vi "Text control 2 v0.7.vi"() -> ()   [LabVIEW 2016]
panel:
  out "error out":errorcluster
  in  "Units":bool
  out "Elapsed Time":dbl caption="Elapsed Time (s)"
  out "Ion vs time":cluster{"Y data in":dbl[], "X data in":dbl[]}[](graph)
  out "Ig":dbl format="%.2e"
  out "Id":dbl format="%.2e"
  out "Is":dbl format="%.2e"
  out "I vs Vg":cluster{"Y data in":dbl[], "X data in":dbl[]}[](graph)
  in  "Panel Controls 2":T1={"Emergency Stop"=refnum, "TransGraph Max"=1e-05, "Text/Graph (text=false)"=TRUE, "TransGraph Min"=1e-11} {"TransGraph Min" format="%.2e"; "TransGraph Max" format="%.2e"}
  out "Currently running:":string="#output s 0 0 0 -0.008 0.008 0.002"
  in  "Lines left to run:":string
  in  "Standby":T2
  in  "Full Reset":bool
  in  "SMU4":cluster{"on/off":bool, "Voltage":dbl} {"Voltage" min=-100.0 max=100.0 format="%.2f"}
  in  "Source/Drain Range":u8(slide)=6 max=11 scale=0.0..11.0
  in  "Source/Drain\nRange mode":u16(ring) items=["Auto", "Limited", "Fixed"]
  in  "Gate Range":u8(slide)=6 max=11 scale=0.0..11.0
  in  "Gate Range\nmode":u16(ring) items=["Auto", "Limited", "Fixed"]
  in  "Gate":T3={"Gate Start"=0.0, "Gate Stop"=2.0, "Gate Step (linear only)"=1.0, "Gate Compliance"=0.0001, "Gate PComp"=0.0, "Range mode"=0, "Range"=6} {"Range" max=11 scale=0.0..11.0; "Range mode" items=["Auto", "Limited", "Fixed"]; "Gate PComp" format="%^.2e"; "Gate Compliance" format="%^.2e"; "Gate Step (linear only)" format="%^.4e"; "Gate Stop" format="%^.4e"; "Gate Start" format="%^.4e"}
  in  "Drain 2":T4={"Drain Start"=0.0, "Drain Stop"=2.0, "Drain Compliance"=0.0001, "Drain Step"=1.0, "Drain PComp"=0.0, "Range mode"=0, "Range"=6} {"Range" max=11 scale=0.0..11.0; "Range mode" items=["Auto", "Limited", "Fixed"]; "Drain PComp" format="%^.2e"; "Drain Step" format="%^.4e"; "Drain Compliance" format="%^.2e"; "Drain Stop" format="%^.4e"; "Drain Start" format="%^.4e"}
  in  "Timings 2":T5={"integration time"=0, "Short/Long integration time"=0.00064, "hold time (sec)"=0.0, "delay time (sec)"=0.0, "Step Time (0 disables)"=0.0, "sweep method"=0, "Pulse period"=0.005, "Base voltage"=0.0, "Pulse width"=0.0005} {"Pulse width" min=0.0005 max=0.1 step=0.0001 format="%.4f"; "Base voltage" format="%^.4e"; "Pulse period" min=0.005 max=1.0 step=0.0001 format="%.4f"; "sweep method" items=["Continuous", "Pulsed"]; "Step Time (0 disables)" format="%.2f"; "delay time (sec)" format="%.4f"; "hold time (sec)" format="%.4f"; "Short/Long integration time" format="%^.0e"; "integration time" scale=0.0..2.0}
  in  "Panel Controls":T6={"Emergency Stop"=refnum, "TransGraph Max"=1e-05, "Text/Graph (text=false)"=TRUE} {"TransGraph Max" format="%.2e"}
  in  "Interrupt run":bool
  in  "Drain: Compliance":dbl=0.001 format="%.8f"
  in  "Gate: Compliance":dbl=0.001 format="%.8f"
  out "Path":path=path "C:/users/rlp38/09Apr2009LTtesting/test2.txt"
  in  "hold time /s":dbl format="%.2f"
  in  "delay time /s":dbl format="%.2f"
  in  "integration time":u32(slide) max=2 step=1 scale=0.0..2.0
  in  "Integration time (short)":dbl=0.0019 min=8e-05 max=0.0019 step=8e-05 format="%^.0e"
  in  "Integration time (long)":dbl=0.32 min=0.04 max=2.0 step=0.02 format="%.2f"
  in  "Step delay /s":dbl format="%.2f"
  in  "Program":string="#pulsedstressV d 0.03 20 0 0.5 0.0827 5\n#\nitime s\ngaterangemode l\ndrainrangemode l\n#pulsed on 0.05 0 0.02\ntransfer d 1 -1 -0.1 -1 -1 0\nwait-min 1\ntransfer d 1 -1 -0.1 -1 -1 0\n#transfer d -10 40 1 5 40 35\n#transfer d -10 40 1 5 40 35\n#output d 0 40 20 0 40 1\n#\n#\n#sample 1 0.008 221 6 0.003\n#samplei 400e-6 200 6 0.002 0.1\n#vsu2pulse -10 4\n#\n#stressV 0.016 0.03 2e-4 0.1e-3 11\n#stressI 220e-7 0.08 15\n#transfer s -1 1 0.5 -0.005 0.005 0.005\n#output s 0 0 0 -0.008 0.008 0.002\n"
  # "Syntax:\nitime [s|m|l]\ngaterangemode [a|l|f]\ndrainrangemode [a|l|f]\npulsed [on|off] PulsePeriod(sec) PulseBaseVoltage PulseONWidth(sec)\nstandby [on l off]\nwait NumMilliseconds\nwait-min NumMinutes\n# texthere = comment\ntransfer [s|d] VgStart VgStop VgStep VdStart VdStop VdStep\noutput [s|d] VgStart VgStop VgStep VdStart VdStop VdStep\nsample Vg Vd NumSamples Time(s) SampleInterval(s)\nsamplei Idg NumSamples Time(s) SampleInterval(s) VDGcompliance\n# if in doubt use SampleInterval(s) = 0.004\nstressV VG VD IGcompliance IDcompliance Duration(sec)\nstressI IDG VDGcompliance Duration(sec)\nvsu2pulse Bias Duration(s)\npulsedstressV [s|d] VEstop VgON VgOFF Period(s) PulseONwidth(s) Vd\nsample-fpp Vg Vd NumSamples Time\nresample-fpp Vg Vd\ntransfer-fpp [s|d] VgStart VgStop VgStep VdStart VdStop VdStep\noutput-fpp [s|d] VgStart VgStop VgStep VdStart VdStop VdStep"
  # "Sec"
  # "Min"
  # "100 samples is approx 13s with medium integration"
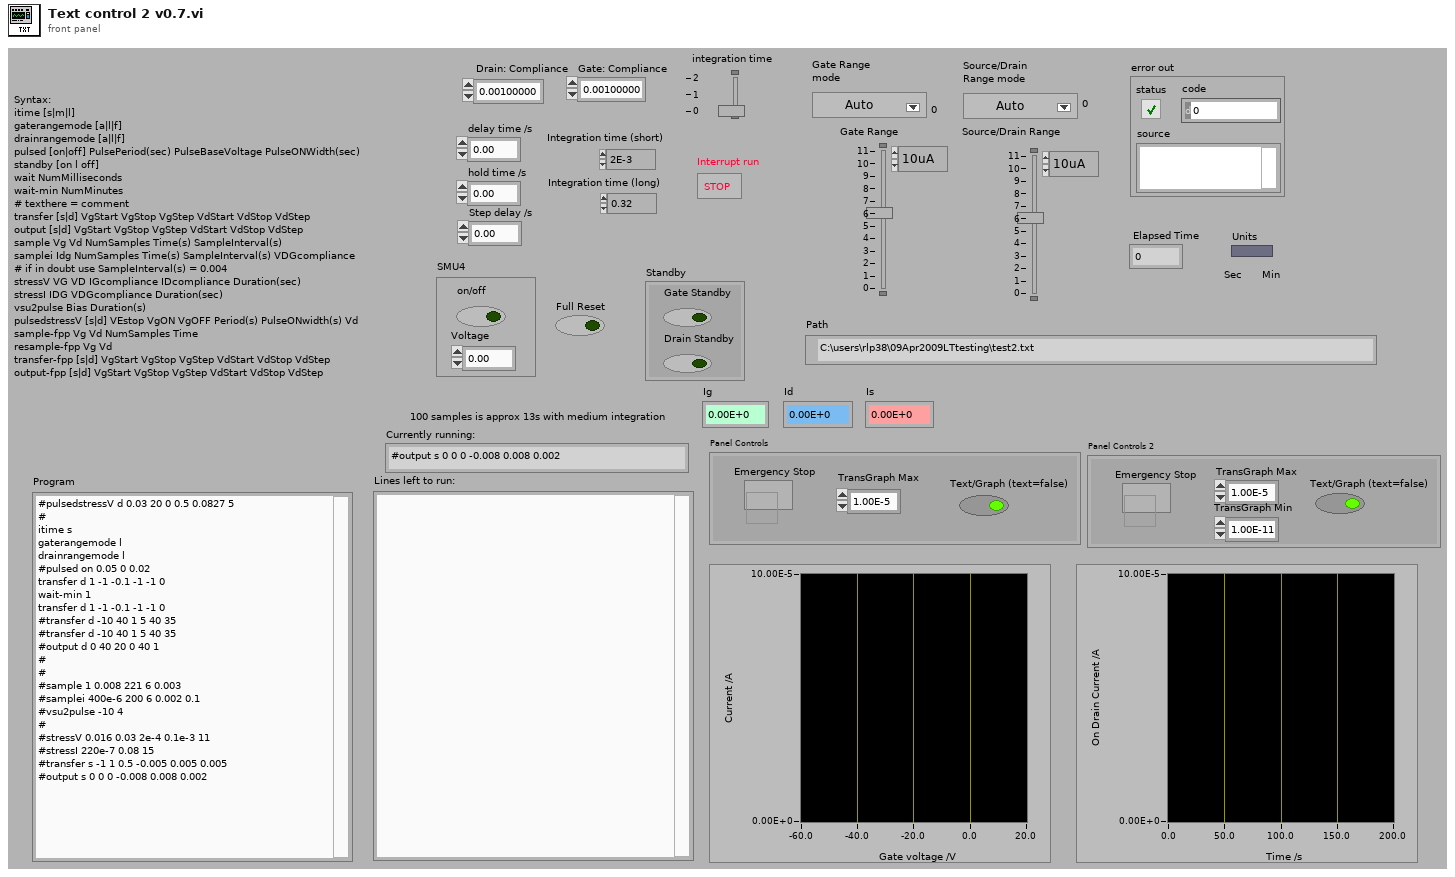
[diagram p1: front panel]
types:
  T1 = cluster{"Emergency Stop":refnum<vi>, "TransGraph Max":dbl, "Text/Graph (text=false)":bool, "TransGraph Min":dbl}
  T2 = cluster{"Gate Standby":bool, "Drain Standby":bool}
  T3 = cluster{"Gate Start":dbl, "Gate Stop":dbl, "Gate Step (linear only)":dbl, "Gate Compliance":dbl, "Gate PComp":dbl, "Range mode":u16, "Range":u8}
  T4 = cluster{"Drain Start":dbl, "Drain Stop":dbl, "Drain Compliance":dbl, "Drain Step":dbl, "Drain PComp":dbl, "Range mode":u16, "Range":u8}
  T5 = cluster{"integration time":u32, "Short/Long integration time":dbl, "hold time (sec)":dbl, "delay time (sec)":dbl, "Step Time (0 disables)":dbl, "sweep method":u16, "Pulse period":dbl, "Base voltage":dbl, "Pulse width":dbl}
  T6 = cluster{"Emergency Stop":refnum<vi>, "TransGraph Max":dbl, "Text/Graph (text=false)":bool}
  T7 = enum16{"open", "replace", "create", "open or create", "replace or create", "replace or create with confirmation"}
  T8 = cluster{"V2 Start":dbl, "V2 Step":dbl, "Number of points":i32}
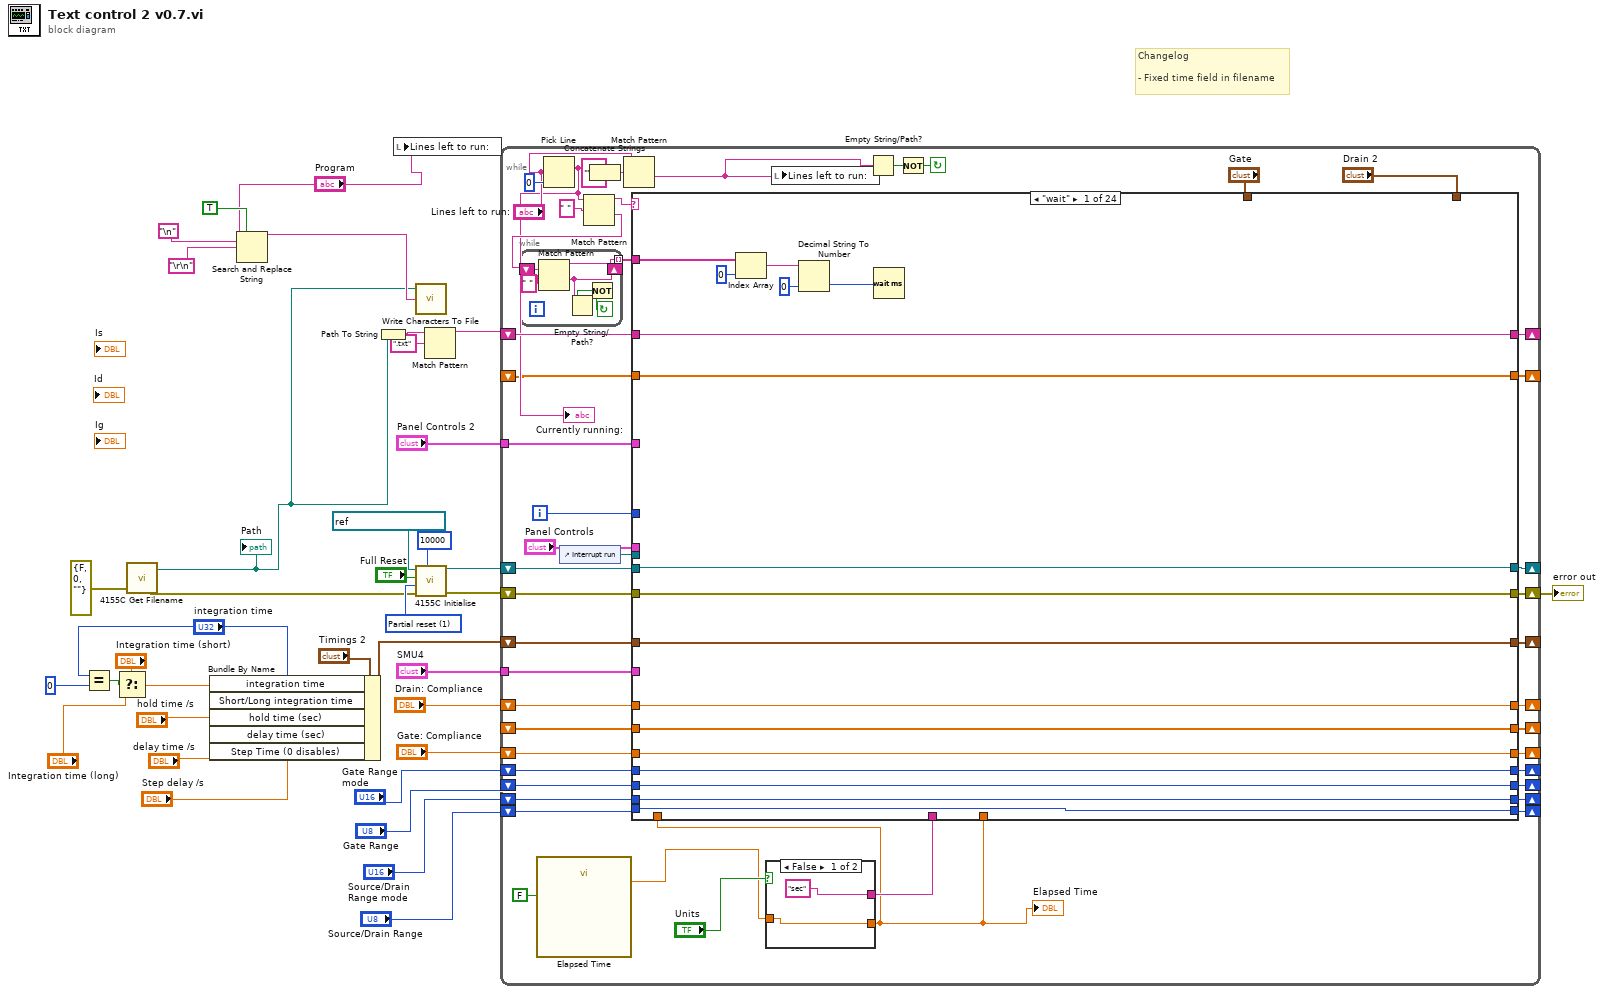
[diagram p0: block diagram]
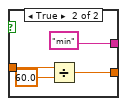
[diagram p2: hidden frame]
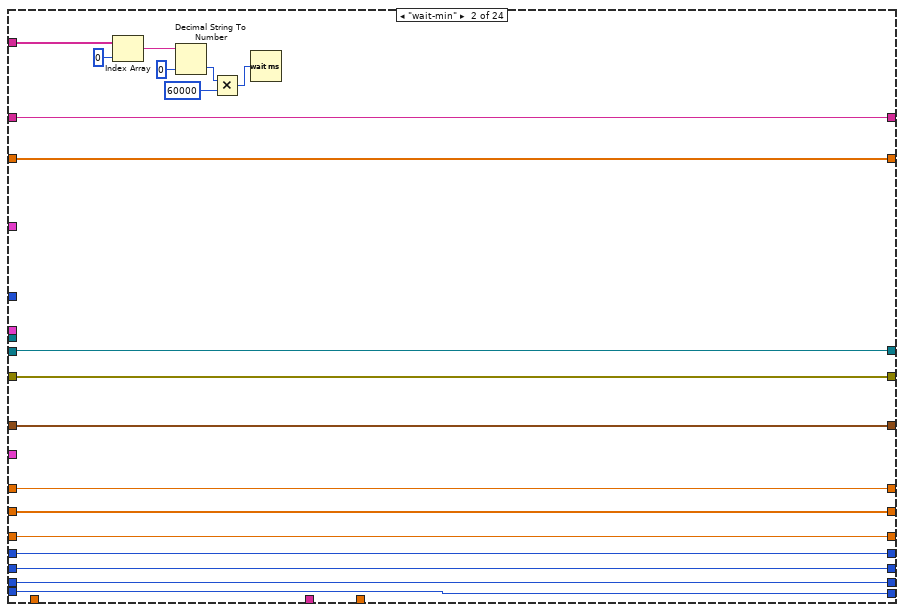
[diagram p3: hidden frame]
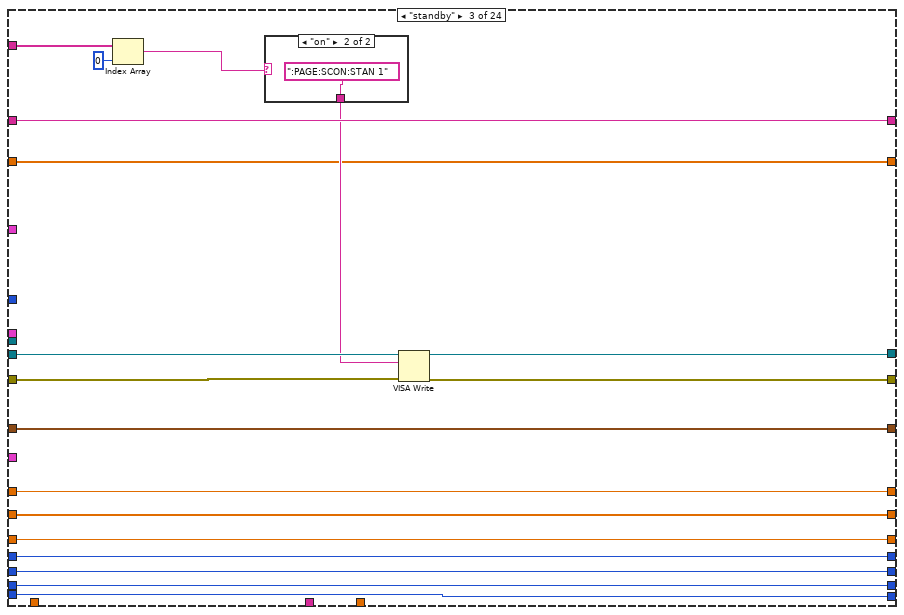
[diagram p4: hidden frame]
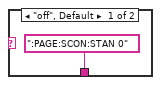
[diagram p5: hidden frame]
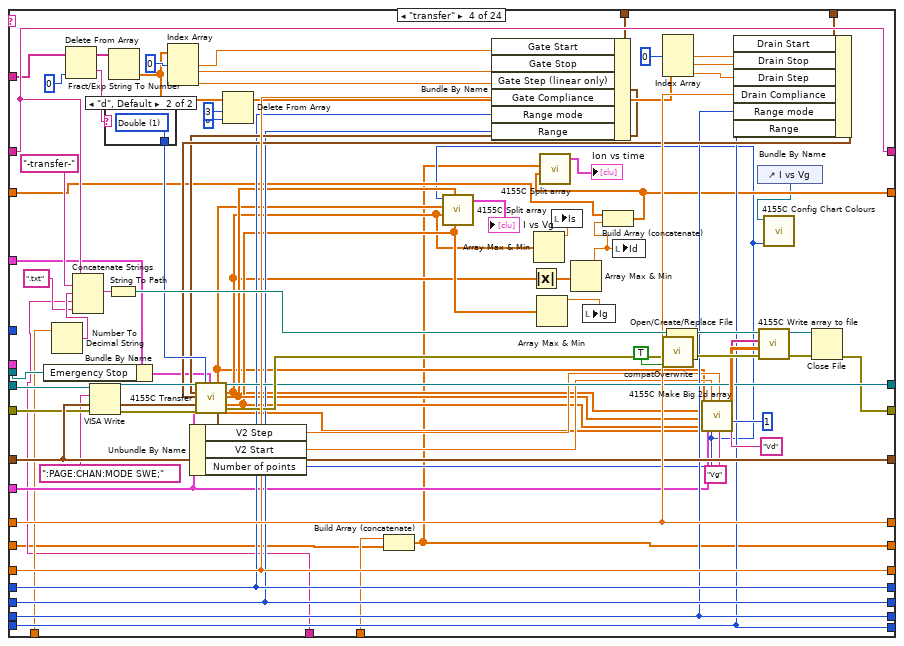
[diagram p6: hidden frame]
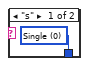
[diagram p7: hidden frame]
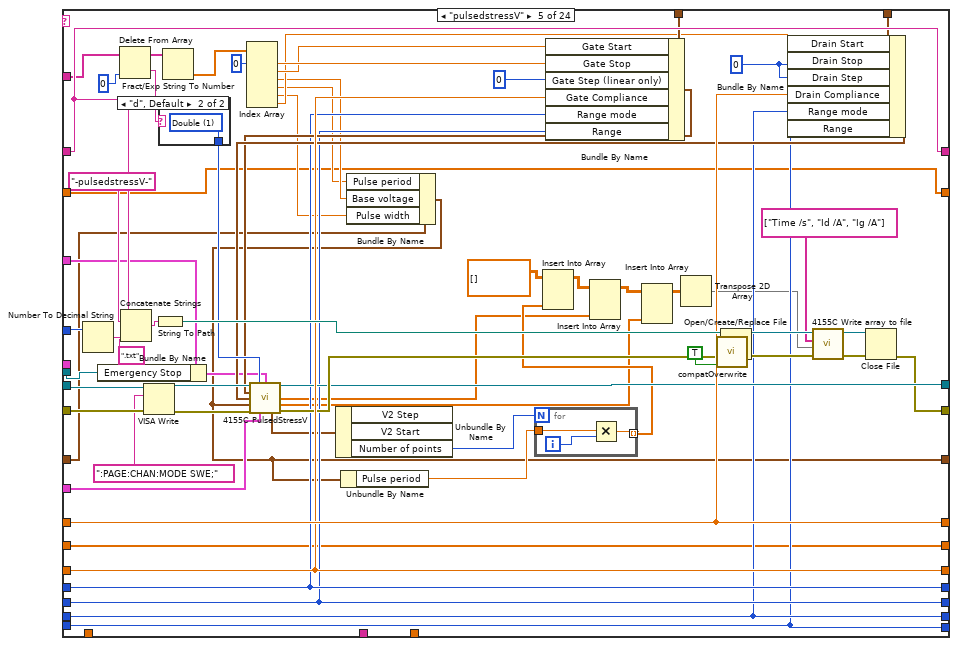
[diagram p8: hidden frame]
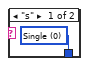
[diagram p9: hidden frame]
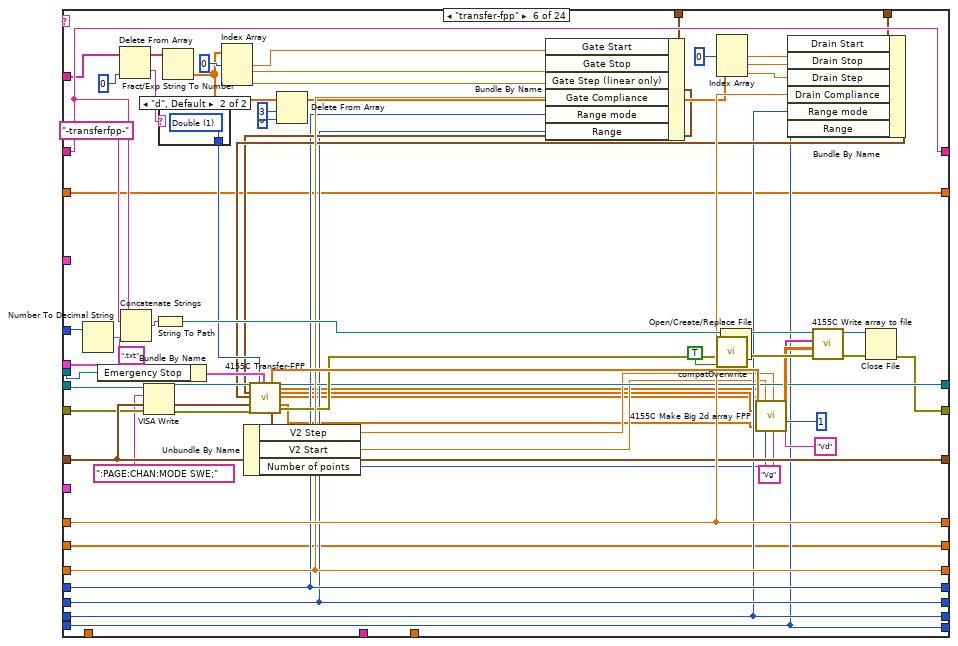
[diagram p10: hidden frame]
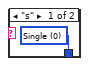
[diagram p11: hidden frame]
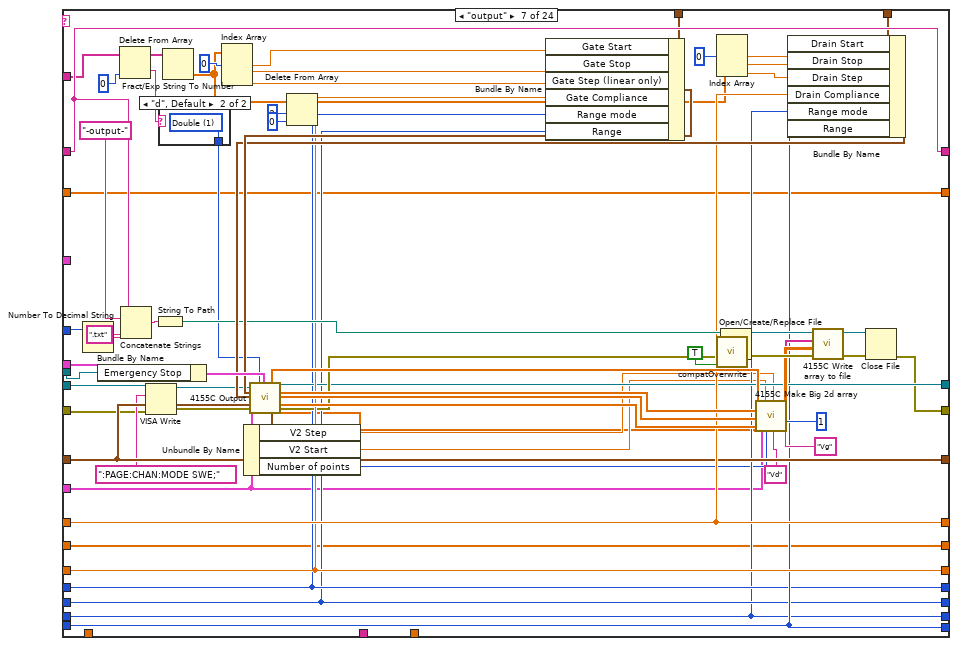
[diagram p12: hidden frame]
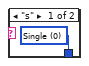
[diagram p13: hidden frame]
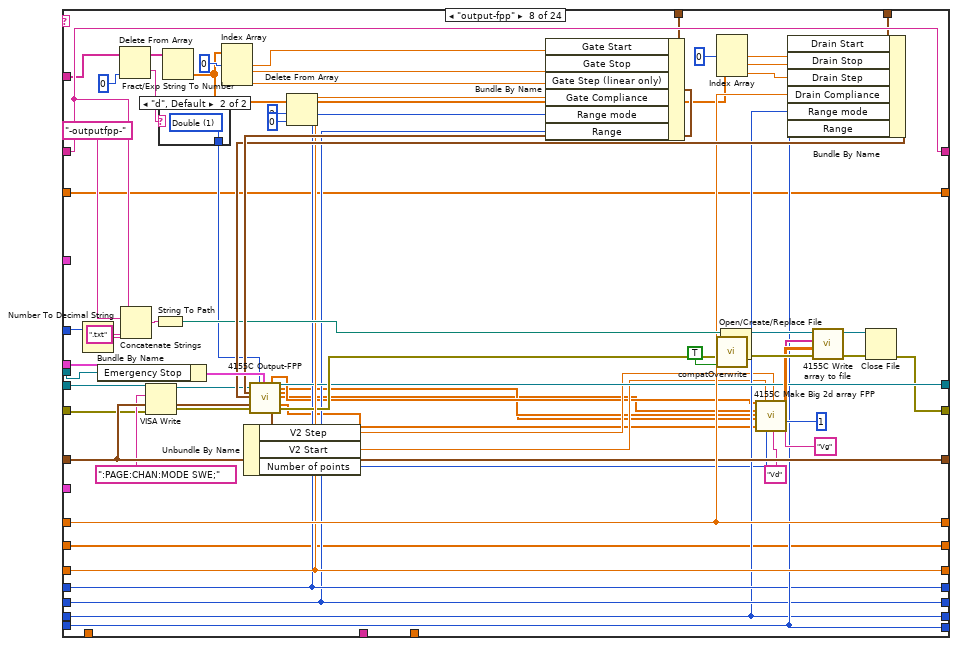
[diagram p14: hidden frame]
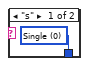
[diagram p15: hidden frame]
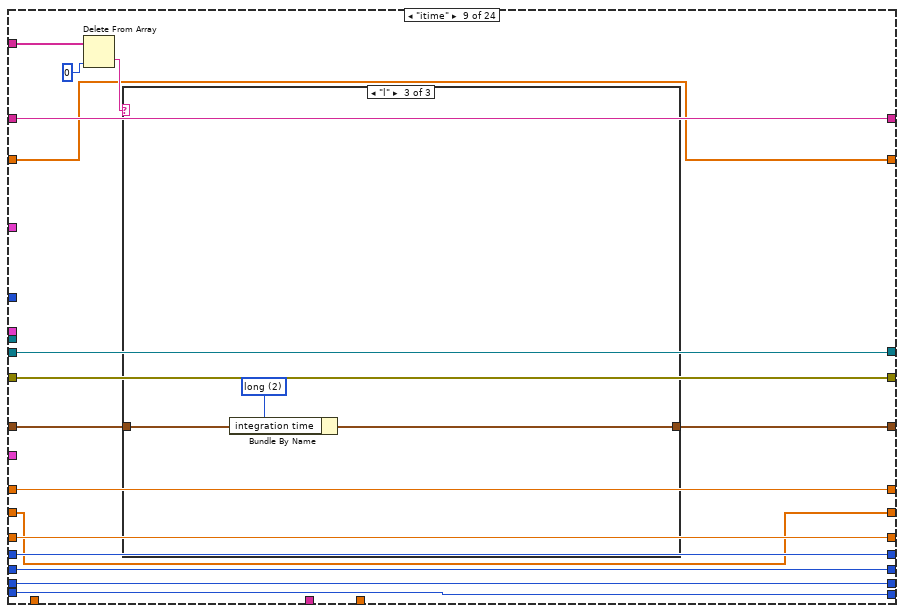
[diagram p16: hidden frame]
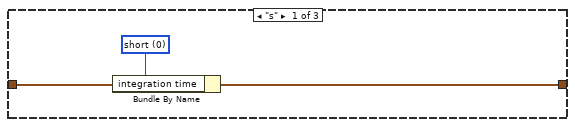
[diagram p17: hidden frame]
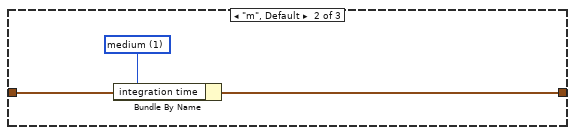
[diagram p18: hidden frame]
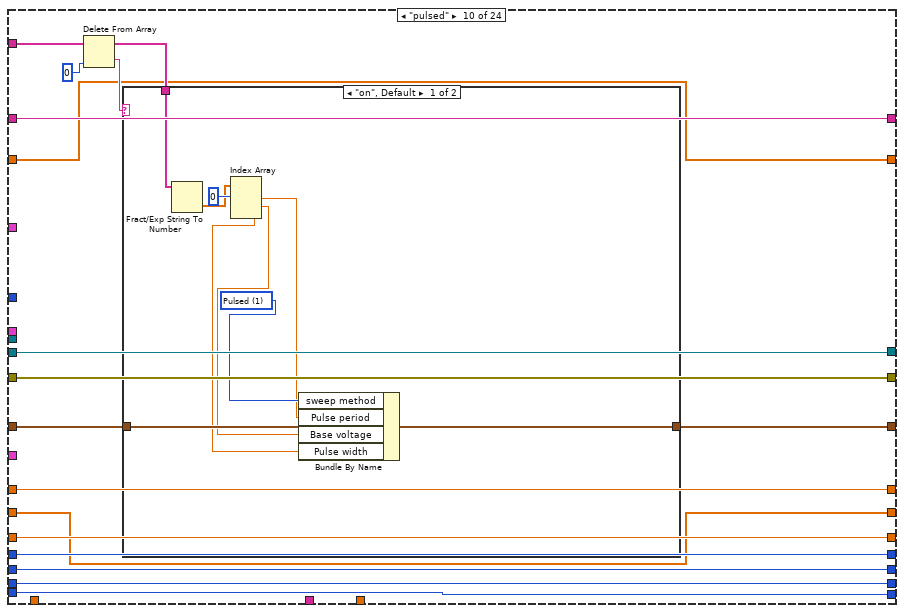
[diagram p19: hidden frame]
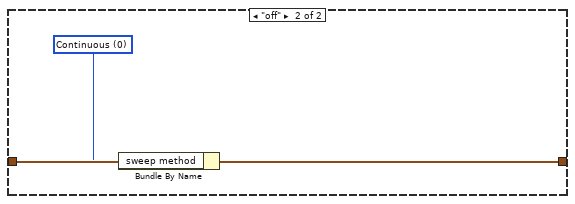
[diagram p20: hidden frame]
diagram:
  w28 = u16 1 items=["Reset All", "Partial reset"] ("Type of reset")
  # "Changelog\n\n- Fixed time field in filename"
  n1 = Equal?(x="integration time", y=u32 0) -> (x = y?=w32:bool)
  n2 = Select(t="Integration time (short)", s=w32, f="Integration time (long)") -> (s? t:f=w36:dbl)
  n3 = call <userlib>:"4155C Get Filename.vi"("error in (no error)"=errorcluster {"status"=FALSE, "code"=0, "source"=""}) -> ("error out"=w23:errorcluster, "path"=w7:path)  [unwired: 2 in, 1 out]
  "Path" <- w7
  n4 = Bundle By Name(cluster="Timings 2", "integration time"="integration time", "Short/Long integration time"=w36, "hold time (sec)"="hold time /s", "delay time (sec)"="delay time /s", "Step Time (0 disables)"="Step delay /s") -> (w20:T5)
  n5 = Search and Replace String(replace all?=TRUE ("replace all? (F)"), input string="Program", search string="\n", replace string="\r\n") -> (result string=w10:string)  [unwired: 4 in, 3 out]
  n6 = Path To String(path=w7) -> (string=w6:string)
  n7 = local write "Lines left to run:"("Program") -> ()
  n8 = call <vilib>:"Write Characters To File.vi"("character string"=w10, "file path (dialog if empty)"=w7) -> ()  [unwired: 3 in, 1 out]
  n9 = call <userlib>:"4155C Initialise.vi"("VISA resource name in"=refnum<visa-resource-name> "GPIB0::14::INSTR", "Reset"="Full Reset", "Type of reset"=w28, "error in (no error)"=w23, "VISA Timeout Value"=u32 10000) -> ("VISA Resource Name out"=w22:refnum<visa-resource-name>, "error out"=w21:errorcluster)
  n10 = Match Pattern(string=w6, regular expression=".txt") -> (before substring=w5:string)  [unwired: 1 in, 3 out]
  n11 = while {
    tunnel: "SMU4" -> [w51]
    shift-left: "Source/Drain Range" -> [w56]
    shift-right: [w52] -> _
    shift-left: "Source/Drain\nRange mode" -> [w57]
    shift-right: [w53] -> _
    shift-left: "Gate Range" -> [w58]
    shift-right: [w54] -> _
    shift-left: "Gate Range\nmode" -> [w59]
    shift-right: [w55] -> _
    shift-left: "Gate: Compliance" -> [w71]
    shift-right: [w65] -> _
    shift-left: "Drain: Compliance" -> [w72]
    shift-right: [w66] -> _
    shift-left: w20 -> [w73]
    shift-right: [w67] -> _
    shift-left: w21 -> [w74]
    shift-right: [w68] -> w1
    shift-left: w22 -> [w75]
    shift-right: [w69] -> _
    shift-left: w5 -> [w76]
    shift-right: [w64] -> _
    tunnel: "Panel Controls 2" -> [w47]
    shift-right: [w46] -> _
    shift-left: _ -> [w45]
    shift-right: [w39] -> _
    shift-left: _ -> [w38]
    i -> [w70]
    stop <- w84 continue-if-true
    n12 = call "Elapsed Time"("Auto Reset"=FALSE) -> ("Elapsed Time (s)"=w41:dbl)  [unwired: 11 in, 7 out]
    n13 = Pick Line(multi-line string="Lines left to run:", line index=0) -> (output string=w48:string)  [unwired: 1 in]
    "Currently running:" <- w48
    n14 = control-ref of="Interrupt run"() -> (w63:refnum<vi>)
    n15 = Match Pattern(string=w48, regular expression=" ") -> (before substring=w79:string, after substring=w78:string)  [unwired: 1 in, 2 out]
    n16 = while {
      tunnel: [w92] -> w77 mode=indexing
      shift-left: w78 -> [w94]
      shift-right: [w93] -> _
      stop <- w96 continue-if-true
      n17 = Match Pattern(string=w94, regular expression=" ") -> (before substring=w92:string, after substring=w93:string)  [unwired: 1 in, 2 out]
      n18 = Empty String/Path?(string/path=w93) -> (empty?=w97:bool)
      n19 = Not(x=w97) -> (.not. x?=w96:bool)
    }
    n20 = Concatenate Strings(w48, "\n" ("Substring")) -> (w82:string)
    n21 = Match Pattern(string="Lines left to run:", regular expression=w82) -> (after substring=w49:string)  [unwired: 1 in, 3 out]
    n22 = case shown="False" "Units" {
      tunnel: ["sec" "min"] -> w42
      tunnel: [w86 w90] -> w40
      tunnel: w41 -> [w86 w89]
      frame False {
      }
      frame True {
        n23 = Divide(x=w89, y=60.0) -> (x/y=w90:dbl)
      }
    }
    "Elapsed Time" <- w40
    n24 = case shown="\"wait\"" w79 {
      tunnel: w77 -> [w114 w133 w151 w215 w284 w352 w418 w492 w531 w557 w584 w609 w630 w644 _ _ w745 w805 _ w869 w912 w953 w1022 w1083]
      tunnel: w76 -> [w109 w129 w149 w223 w291 w360 w426 w500 w520 w546 w576 w602 w624 w637 w656 w696 w723 w787 w819 w856 w899 w941 w1016 w1079]
      tunnel: w75 -> [w108 w128 w140 w193 w275 w329 w394 w468 w521 w547 w577 w603 w625 w638 w661 w699 w752 w812 w823 w876 w919 w960 w1029 w1036]
      tunnel: w74 -> [w107 w127 w139 w192 w274 w328 w391 w465 w522 w548 w578 w604 w626 w639 w660 w668 w751 w811 w822 w875 w918 w959 w1028 w1035]
      tunnel: w73 -> [w106 w126 w148 w219 w249 w356 w422 w496 w530 w556 w575 w601 w623 w636 w659 w692 w714 w779 w828 w849 w892 w934 w1015 w1078]
      tunnel: w72 -> [w105 w125 w147 w221 w289 w358 w424 w498 w529 w555 w583 w608 w629 w643 w658 w677 w750 w810 w831 w874 w917 w958 w1027 w1088]
      tunnel: w71 -> [w104 w124 w146 w220 w288 w357 w423 w497 w528 w554 w582 w607 w628 w642 w657 w678 w724 w788 w830 w857 w900 w942 w1017 w1080]
      tunnel: w70 -> [_ _ _ _ w292 w361 w427 w501 _ _ _ _ _ _ _ w694 w749 w809 _ w873 w916 w957 w1026 w1087]
      tunnel: [w108 w128 w138 w217 w286 w354 w420 w494 w521 w547 w577 w603 w625 w638 w661 w699 w715 w760 w821 w850 w893 w935 w967 w1038] -> w69
      tunnel: [w107 w127 w137 w216 w285 w353 w419 w493 w522 w548 w578 w604 w626 w639 w660 w667 w725 w761 w820 w858 w901 w943 w966 w1037] -> w68
      tunnel: [w106 w126 w148 w219 w245 w356 w422 w496 w523 w549 w575 w601 w623 w636 w659 w692 w714 w779 w828 w849 w892 w934 w1015 w1078] -> w67
      tunnel: [w105 w125 w147 w221 w289 w358 w424 w498 w529 w555 w583 w608 w629 w643 w658 w677 w750 w810 w831 w874 w917 w958 w1027 w1088] -> w66
      tunnel: [w104 w124 w146 w220 w288 w357 w423 w497 w528 w554 w582 w607 w628 w642 w657 w678 w724 w788 w830 w857 w900 w942 w1017 w1080] -> w65
      tunnel: [w109 w129 w149 w223 w291 w360 w426 w500 w520 w546 w576 w602 w624 w637 w656 w696 w723 w787 w819 w856 w899 w941 w1016 w1079] -> w64
      tunnel: w63 -> [_ _ _ w226 w296 w366 w435 w505 _ _ _ _ _ _ _ _ w720 w784 _ w855 w898 w940 w987 w1054]
      tunnel: "Gate" -> [_ _ _ w202 w278 w339 w405 w479 _ _ _ _ _ _ _ _ _ _ _ _ _ _ _ _]
      tunnel: "Drain 2" -> [_ _ _ w201 w277 w338 w404 w478 _ _ _ _ _ _ _ _ _ _ _ _ _ _ _ _]
      tunnel: "Panel Controls" -> [_ _ _ _ _ w337 w403 w477 _ _ _ _ _ _ _ _ _ _ _ _ _ _ _ _]
      tunnel: w59 -> [w103 w123 w145 w186 w268 w322 w389 w463 w527 w553 _ w600 w622 w635 w655 w679 w710 w775 w824 w845 w888 w930 w1011 w1074]
      tunnel: w58 -> [w102 w122 w144 w185 w267 w321 w388 w462 w526 w552 w581 _ w613 w641 w654 w680 w711 w776 w825 w846 w889 w931 w1012 w1075]
      tunnel: w57 -> [w101 w121 w143 w184 w266 w320 w387 w461 w525 w551 w580 w606 w627 _ w653 w681 w712 w777 w826 w847 w890 w932 w1013 w1076]
      tunnel: w56 -> [w100 w120 w142 w183 w265 w319 w390 w464 w524 w550 w579 w605 _ w640 w652 w682 w713 w778 w827 w848 w891 w933 w1014 w1077]
      tunnel: [w103 w123 w145 w186 w268 w322 w389 w463 w527 w553 w574 w600 w622 w635 w655 w679 w710 w775 w824 w845 w888 w930 w1011 w1074] -> w55
      tunnel: [w102 w122 w144 w185 w267 w321 w388 w462 w526 w552 w581 w592 w613 w641 w654 w680 w711 w776 w825 w846 w889 w931 w1012 w1075] -> w54
      tunnel: [w101 w121 w143 w184 w266 w320 w387 w461 w525 w551 w580 w606 w627 w634 w653 w681 w712 w777 w826 w847 w890 w932 w1013 w1076] -> w53
      tunnel: [w100 w120 w142 w183 w265 w319 w390 w464 w524 w550 w579 w605 w614 w640 w652 w682 w713 w778 w827 w848 w891 w933 w1014 w1077] -> w52
      tunnel: w51 -> [_ _ _ w178 w261 _ w381 _ _ _ _ _ _ _ _ _ _ _ _ _ _ _ _ _]
      tunnel: w47 -> [_ _ _ w176 w260 _ _ _ _ _ _ _ _ _ _ _ _ _ _ _ _ _ _ _]
      tunnel: [w99 w116 w135 w165 w237 w308 w378 w449 w519 w544 w573 w591 w612 w633 w651 w663 w701 w758 w818 w833 w880 w923 w964 w1031] -> w46
      tunnel: w45 -> [w99 w116 w135 w164 w237 w308 w378 w449 w519 w544 w573 w591 w612 w633 w651 w663 w701 w758 w818 w833 w880 w923 w964 w1031]
      tunnel: w40 -> [_ _ _ w160 _ _ _ _ _ _ _ _ _ _ _ _ _ _ _ _ _ _ _ _]
      tunnel: w42 -> [_ _ _ w157 _ _ _ _ _ _ _ _ _ _ _ _ _ _ _ _ _ _ _ _]
      tunnel: w40 -> [_ _ _ w156 _ _ _ _ _ _ _ _ _ _ _ _ _ _ _ _ _ _ _ _]
      tunnel: [w98 w115 w134 w154 w236 w307 w377 w448 w518 w543 w572 w590 w611 w632 w650 w662 w700 w757 w817 w832 w879 w922 w963 w1030] -> w39
      tunnel: w38 -> [w98 w115 w134 w155 w236 w307 w377 w448 w518 w543 w572 w590 w611 w632 w650 w662 w700 w757 w817 w832 w879 w922 w963 w1030]
      frame "wait" {
        n25 = Index Array(array=w114, index=0 ("Index")) -> (element=w112:string)
        n26 = Decimal String To Number(string=w112, default (0L)=u32 0) -> (number=w111:u32)  [unwired: 1 in, 1 out]
        n27 = Wait (ms)(milliseconds to wait=w111) -> ()  [unwired: 1 out]
      }
      frame "wait-min" {
        n28 = Index Array(array=w133, index=0 ("Index")) -> (element=w131:string)
        n29 = Decimal String To Number(string=w131, default (0L)=u32 0) -> (number=w119:u32)  [unwired: 1 in, 1 out]
        n30 = Multiply(x=w119, y=u32 60000) -> (x*y=w118:u32)
        n31 = Wait (ms)(milliseconds to wait=w118) -> ()  [unwired: 1 out]
      }
      frame "standby" {
        n32 = Index Array(array=w151, index=0 ("Index")) -> (element=w141:string)
        n33 = case shown="\"on\"" w141 {
          tunnel: [":PAGE:SCON:STAN 0" ":PAGE:SCON:STAN 1"] -> w136
          frame "off", Default {
          }
          frame "on" {
          }
        }
        n34 = VISA Write(VISA resource name=w140, write buffer=w136, error in (no error)=w139) -> (VISA resource name out=w138:refnum<visa-resource-name>, error out=w137:errorcluster)  [unwired: 1 out]
      }
      frame "transfer" {
        n35 = Bundle By Name(cluster=w176, "Emergency Stop"=w226) -> (w177:T1)
        n36 = Number To Decimal String(number=w160) -> (decimal integer string=w159:string)  [unwired: 1 in]
        n37 = Delete From Array(array=w215, index=0 ("Index")) -> (deleted portion=w213:string, array with subset deleted=w212:string[])  [unwired: 1 in]
        n38 = Concatenate Strings(w223, "-transfer-" ("Prefix"), w159, w157, ".txt" ("Suffix")) -> (w225:string)
        n39 = VISA Write(VISA resource name=w193, write buffer=":PAGE:CHAN:MODE SWE;" ("write buffer (\"\")"), error in (no error)=w192) -> (VISA resource name out=w190:refnum<visa-resource-name>, error out=w191:errorcluster)  [unwired: 1 out]
        n40 = case shown="\"d\", Default" w213 {
          tunnel: [w234 w235] -> w211
          frame "s" {
            w234 = u16 0 items=["Single", "Double"] ("sweep mode")
          }
          frame "d", Default {
            w235 = u16 1 items=["Single", "Double"] ("sweep mode")
          }
        }
        n41 = String To Path(string=w225) -> (path=w222:path)
        n42 = Fract/Exp String To Number(string=w212) -> (number=w197:dbl[])  [unwired: 3 in, 1 out]
        n43 = Index Array(array=w197, index #1=0 ("Index")) -> (element #1=w210:dbl, element #2=w209:dbl, element #3=w208:dbl)  [unwired: 2 in]
        n44 = Delete From Array(array=w197, length=3 ("Length"), index=0 ("Index")) -> (array with subset deleted=w195:dbl[])  [unwired: 1 out]
        n45 = Build Array (concatenate)(w156, w155) -> (w154:dbl[])
        n46 = Bundle By Name(cluster=w202, "Gate Start"=w210, "Gate Stop"=w209, "Gate Step (linear only)"=w208, "Gate Compliance"=w220, "Range mode"=w186, "Range"=w185) -> (w187:T3)
        n47 = Index Array(array=w195, index #1=0 ("Index")) -> (element #1=w205:dbl, element #2=w204:dbl, element #3=w203:dbl)  [unwired: 2 in]
        n48 = call <vilib>:"compatOverwrite.vi"("overwrite (F)"=TRUE) -> ("overwrite?"=w175:T7)
        n49 = Bundle By Name(cluster=w201, "Drain Start"=w205, "Drain Stop"=w204, "Drain Step"=w203, "Drain Compliance"=w221, "Range mode"=w184, "Range"=w183) -> (w188:T4)
        n50 = call <userlib>:"4155C Transfer.vi"("VISA resource name in"=w190, "Gate"=w187, "Drain"=w188, "Timings"=w219, "error in (no error)"=w191, "SMU4"=w178, "sweep mode"=w211, "Panel Controls"=w177) -> ("VG"=w166:dbl[], "Outparams"=w182:T8, "VISA Resource Name out"=w217:refnum<visa-resource-name>, "IS"=w168:dbl[], "ID"=w173:dbl[], "IG"=w169:dbl[], "error out"=w218:errorcluster, "SMU4"=w179:dbl[])  [unwired: 12 in]
        n51 = Unbundle By Name(w182) -> ("V2 Step"=w181:dbl, "V2 Start"=w180:dbl, "Number of points"=w162:i32)
        n52 = call <userlib>:"4155C Split array.vi"("Number of VAR2 steps"=w162, "Y2 data in"=w173, "X data in"=w166, "Y1 data in"=w168, "Y3 data in"=w169) -> ("Array of clusters"=→"I vs Vg":cluster{"Y data in":dbl[], "X data in":dbl[]}[])  [unwired: 2 in, 1 out]
        n53 = Absolute Value(x=w168) -> (abs(x)=w172:dbl[])
        n54 = Array Max & Min(array=w168) -> (max value=w170:dbl)  [unwired: 3 out]
        n55 = Array Max & Min(array=w169) -> (max value=w171:dbl)  [unwired: 3 out]
        n56 = local write "Is"(w170) -> ()
        n57 = Array Max & Min(array=w172) -> (max value=w163:dbl)  [unwired: 3 out]
        n58 = local write "Ig"(w171) -> ()
        n59 = Build Array (concatenate)(w164, w163) -> (w165:dbl[])
        n60 = call <userlib>:"4155C Split array.vi"("X data in"=w154, "Y1 data in"=w165) -> ("Array of clusters"=→"Ion vs time":cluster{"Y data in":dbl[], "X data in":dbl[]}[])  [unwired: 5 in, 1 out]
        n61 = local write "Id"(w163) -> ()
        n62 = Open/Create/Replace File(file path (use dialog)=w222, error in=w218, operation (0:open)=w175) -> (refnum out=w231:refnum<file>, error out=w232:errorcluster)  [unwired: 3 in, 1 out]
        n63 = call <userlib>:"4155C Make Big 2d array.vi"("1D Var1"=w166, "1d IS"=w168, "1d ID"=w173, "1d IG"=w169, "1d SMU4"=w179, "SMU4"=w178, "VAR2 START"=w180, "Number of VAR2 steps"=w162, "VAR2 STEP"=w181, "VAR1 Name"="Vg", "Decimal places in header"=i8 1, "VAR2 Name"="Vd") -> ("Header array"=w227:string[], "Data array"=w228:dbl[][])  [unwired: 14 in]
        n64 = control-ref of="I vs Vg"() -> (w161:refnum<vi>)
        n65 = call <userlib>:"4155C Write array to file.vi"("Byte Stream File Refnum"=w231, "Header"=w227, "Data Array"=w228, "error in (no error)"=w232) -> ("dup refnum"=w229:refnum<file>, "error out"=w230:errorcluster)  [unwired: 1 in]
        n66 = call <userlib>:"4155C Config Chart Colours.vi"("Numeric"=w162, "XY Graph 2"=w161) -> ()  [unwired: 6 in]
        n67 = Close File(refnum=w229, error in=w230) -> (error out=w216:errorcluster)  [unwired: 1 out]
      }
      frame "pulsedstressV" {
        w243 = 0
        n68 = Number To Decimal String(number=w292) -> (decimal integer string=w293:string)  [unwired: 1 in]
        n69 = Bundle By Name(cluster=w260, "Emergency Stop"=w296) -> (w262:T1)
        n70 = Delete From Array(array=w284, index=0 ("Index")) -> (deleted portion=w282:string, array with subset deleted=w281:string[])  [unwired: 1 in]
        n71 = Concatenate Strings(w291, "-pulsedstressV-" ("Substring"), w293, ".txt" ("Substring")) -> (w295:string)
        n72 = VISA Write(VISA resource name=w275, write buffer=":PAGE:CHAN:MODE SWE;" ("write buffer (\"\")"), error in (no error)=w274) -> (VISA resource name out=w272:refnum<visa-resource-name>, error out=w273:errorcluster)  [unwired: 1 out]
        n73 = String To Path(string=w295) -> (path=w290:path)
        n74 = case shown="\"d\", Default" w282 {
          tunnel: [w305 w306] -> w280
          frame "s" {
            w305 = u16 0 items=["Single", "Double"] ("sweep mode")
          }
          frame "d", Default {
            w306 = u16 1 items=["Single", "Double"] ("sweep mode")
          }
        }
        n75 = Fract/Exp String To Number(string=w281) -> (number=w276:dbl[])  [unwired: 3 in, 1 out]
        n76 = Index Array(array=w276, index #1=0 ("Index")) -> (element #1=w252:dbl, element #2=w251:dbl, element #3=w248:dbl, element #4=w247:dbl, element #5=w246:dbl, element #6=w250:dbl)  [unwired: 5 in]
        n77 = Bundle By Name(cluster=w249, "Pulse period"=w247, "Base voltage"=w248, "Pulse width"=w246) -> (w245:T5)
        n78 = Unbundle By Name(w245) -> ("Pulse period"=w253:dbl)
        n79 = Bundle By Name(cluster=w278, "Gate Start"=w251, "Gate Stop"=w252, "Gate Step (linear only)"=0, "Gate Compliance"=w288, "Range mode"=w268, "Range"=w267) -> (w269:T3)
        n80 = call <vilib>:"compatOverwrite.vi"("overwrite (F)"=TRUE) -> ("overwrite?"=w238:T7)
        n81 = Bundle By Name(cluster=w277, "Drain Start"=w250, "Drain Stop"=w243, "Drain Step"=w243, "Drain Compliance"=w289, "Range mode"=w266, "Range"=w265) -> (w270:T4)
        n82 = call <userlib>:"4155C PulsedStressV.vi"("VISA resource name in"=w272, "sweep mode"=w280, "Panel Controls"=w262, "Gate"=w269, "Drain"=w270, "Timings"=w245, "error in (no error)"=w273, "SMU4"=w261) -> ("VISA Resource Name out"=w286:refnum<visa-resource-name>, "ID"=w241:dbl[], "IG"=w239:dbl[], "Outparams"=w263:T8, "error out"=w287:errorcluster)  [unwired: 3 in]
        n83 = Unbundle By Name(w263) -> ("Number of points"=w240:i32)  [unwired: 2 out]
        n84 = for {
          N: w240 -> [_]
          tunnel: [w302] -> w242 mode=indexing
          tunnel: w253 -> [w304]
          i -> [w303]
          n85 = Multiply(x=w304, y=w303) -> (x*y=w302:dbl)
        }
        n86 = Insert Into Array(array=dbl[][] [] ("Input Array"), new element=w242) -> (w254:dbl[][])  [unwired: 2 in]
        n87 = Insert Into Array(array=w254, new element=w241) -> (w259:dbl[][])  [unwired: 2 in]
        n88 = Insert Into Array(array=w259, new element=w239) -> (w258:dbl[][])  [unwired: 2 in]
        n89 = Transpose 2D Array(2D array=w258) -> (transposed array=w257:dbl[][])
        n90 = Open/Create/Replace File(file path (use dialog)=w290, error in=w287, operation (0:open)=w238) -> (refnum out=w299:refnum<file>, error out=w300:errorcluster)  [unwired: 3 in, 1 out]
        n91 = call <userlib>:"4155C Write array to file.vi"("Byte Stream File Refnum"=w299, "Header"=string[] ["Time /s", "Id /A", "Ig /A"], "Data Array"=w257, "error in (no error)"=w300) -> ("dup refnum"=w297:refnum<file>, "error out"=w298:errorcluster)  [unwired: 1 in]
        n92 = Close File(refnum=w297, error in=w298) -> (error out=w285:errorcluster)  [unwired: 1 out]
      }
      frame "transfer-fpp" {
        n93 = Number To Decimal String(number=w361) -> (decimal integer string=w362:string)  [unwired: 1 in]
        n94 = Bundle By Name(cluster=w337, "Emergency Stop"=w366) -> (w374:T6)
        n95 = Delete From Array(array=w352, index=0 ("Index")) -> (deleted portion=w350:string, array with subset deleted=w349:string[])  [unwired: 1 in]
        n96 = Concatenate Strings(w360, "-transferfpp-" ("Substring"), w362, ".txt" ("Substring")) -> (w364:string)
        n97 = VISA Write(VISA resource name=w329, write buffer=":PAGE:CHAN:MODE SWE;" ("write buffer (\"\")"), error in (no error)=w328) -> (VISA resource name out=w326:refnum<visa-resource-name>, error out=w327:errorcluster)  [unwired: 1 out]
        n98 = String To Path(string=w364) -> (path=w359:path)
        n99 = case shown="\"d\", Default" w350 {
          tunnel: [w375 w376] -> w348
          frame "s" {
            w375 = u16 0 items=["Single", "Double"] ("sweep mode")
          }
          frame "d", Default {
            w376 = u16 1 items=["Single", "Double"] ("sweep mode")
          }
        }
        n100 = Fract/Exp String To Number(string=w349) -> (number=w333:dbl[])  [unwired: 3 in, 1 out]
        n101 = Index Array(array=w333, index #1=0 ("Index")) -> (element #1=w347:dbl, element #2=w346:dbl, element #3=w345:dbl)  [unwired: 2 in]
        n102 = Delete From Array(array=w333, length=3 ("Length"), index=0 ("Index")) -> (array with subset deleted=w331:dbl[])  [unwired: 1 out]
        n103 = Bundle By Name(cluster=w339, "Gate Start"=w347, "Gate Stop"=w346, "Gate Step (linear only)"=w345, "Gate Compliance"=w357, "Range mode"=w322, "Range"=w321) -> (w323:T3)
        n104 = Index Array(array=w331, index #1=0 ("Index")) -> (element #1=w342:dbl, element #2=w341:dbl, element #3=w340:dbl)  [unwired: 2 in]
        n105 = call <vilib>:"compatOverwrite.vi"("overwrite (F)"=TRUE) -> ("overwrite?"=w309:T7)
        n106 = Bundle By Name(cluster=w338, "Drain Start"=w342, "Drain Stop"=w341, "Drain Step"=w340, "Drain Compliance"=w358, "Range mode"=w320, "Range"=w319) -> (w324:T4)
        n107 = call <userlib>:"4155C Transfer-FPP.vi"("VISA resource name in"=w326, "Gate"=w323, "Drain"=w324, "Timings"=w356, "error in (no error)"=w327, "sweep mode"=w348, "Panel Controls"=w374) -> ("VG"=w365:dbl[], "Outparams"=w317:T8, "VISA Resource Name out"=w354:refnum<visa-resource-name>, "Vprobe2"=w313:dbl[], "ID"=w312:dbl[], "IG"=w311:dbl[], "Vprobe1"=w310:dbl[], "error out"=w355:errorcluster)  [unwired: 13 in]
        n108 = Unbundle By Name(w317) -> ("V2 Step"=w316:dbl, "V2 Start"=w315:dbl, "Number of points"=w314:i32)
        n109 = Open/Create/Replace File(file path (use dialog)=w359, error in=w355, operation (0:open)=w309) -> (refnum out=w371:refnum<file>, error out=w372:errorcluster)  [unwired: 3 in, 1 out]
        n110 = call <userlib>:"4155C Make Big 2d array FPP.vi"("1D Var1"=w365, "1d ID"=w312, "1d Vp2"=w313, "1d IG"=w311, "1d Vp1"=w310, "VAR2 START"=w315, "Number of VAR2 steps"=w314, "VAR2 STEP"=w316, "VAR1 Name"="Vg", "Decimal places in header"=i8 1, "VAR2 Name"="Vd") -> ("Header array"=w367:string[], "Data array"=w368:dbl[][])  [unwired: 15 in]
        n111 = call <userlib>:"4155C Write array to file.vi"("Byte Stream File Refnum"=w371, "Header"=w367, "Data Array"=w368, "error in (no error)"=w372) -> ("dup refnum"=w369:refnum<file>, "error out"=w370:errorcluster)  [unwired: 1 in]
        n112 = Close File(refnum=w369, error in=w370) -> (error out=w353:errorcluster)  [unwired: 1 out]
      }
      frame "output" {
        n113 = Number To Decimal String(number=w427) -> (decimal integer string=w428:string)  [unwired: 1 in]
        n114 = Bundle By Name(cluster=w403, "Emergency Stop"=w435) -> (w445:T6)
        n115 = Delete From Array(array=w418, index=0 ("Index")) -> (deleted portion=w416:string, array with subset deleted=w415:string[])  [unwired: 1 in]
        n116 = Concatenate Strings(w426, "-output-" ("Substring"), w428, ".txt" ("Substring")) -> (w430:string)
        n117 = VISA Write(VISA resource name=w394, write buffer=":PAGE:CHAN:MODE SWE;" ("write buffer (\"\")"), error in (no error)=w391) -> (VISA resource name out=w393:refnum<visa-resource-name>, error out=w392:errorcluster)  [unwired: 1 out]
        n118 = String To Path(string=w430) -> (path=w425:path)
        n119 = case shown="\"d\", Default" w416 {
          tunnel: [w446 w447] -> w414
          frame "s" {
            w446 = u16 0 items=["Single", "Double"] ("sweep mode")
          }
          frame "d", Default {
            w447 = u16 1 items=["Single", "Double"] ("sweep mode")
          }
        }
        n120 = Fract/Exp String To Number(string=w415) -> (number=w397:dbl[])  [unwired: 3 in, 1 out]
        n121 = Index Array(array=w397, index #1=0 ("Index")) -> (element #1=w413:dbl, element #2=w412:dbl, element #3=w411:dbl)  [unwired: 2 in]
        n122 = Delete From Array(array=w397, length=3 ("Length"), index=0 ("Index")) -> (array with subset deleted=w396:dbl[])  [unwired: 1 out]
        n123 = Bundle By Name(cluster=w405, "Gate Start"=w413, "Gate Stop"=w412, "Gate Step (linear only)"=w411, "Gate Compliance"=w423, "Range mode"=w389, "Range"=w388) -> (w444:T3)
        n124 = Index Array(array=w396, index #1=0 ("Index")) -> (element #1=w408:dbl, element #2=w407:dbl, element #3=w406:dbl)  [unwired: 2 in]
        n125 = call <vilib>:"compatOverwrite.vi"("overwrite (F)"=TRUE) -> ("overwrite?"=w379:T7)
        n126 = Bundle By Name(cluster=w404, "Drain Start"=w408, "Drain Stop"=w407, "Drain Step"=w406, "Drain Compliance"=w424, "Range mode"=w387, "Range"=w390) -> (w443:T4)
        n127 = call <userlib>:"4155C Output.vi"("VISA resource name in"=w393, "Gate"=w444, "Drain"=w443, "Timings"=w422, "error in (no error)"=w392, "SMU4"=w381, "sweep mode"=w414, "Panel controls"=w445) -> ("VD"=w431:dbl[], "Outparams"=w384:T8, "VISA Resource Name out"=w420:refnum<visa-resource-name>, "IS"=w434:dbl[], "ID"=w433:dbl[], "IG"=w432:dbl[], "error out"=w421:errorcluster, "SMU4"=w380:dbl[])  [unwired: 12 in]
        n128 = Unbundle By Name(w384) -> ("V2 Step"=w385:dbl, "V2 Start"=w383:dbl, "Number of points"=w382:i32)
        n129 = Open/Create/Replace File(file path (use dialog)=w425, error in=w421, operation (0:open)=w379) -> (refnum out=w440:refnum<file>, error out=w441:errorcluster)  [unwired: 3 in, 1 out]
        n130 = call <userlib>:"4155C Make Big 2d array.vi"("1D Var1"=w431, "1d IS"=w434, "1d ID"=w433, "1d IG"=w432, "1d SMU4"=w380, "SMU4"=w381, "VAR2 START"=w383, "Number of VAR2 steps"=w382, "VAR2 STEP"=w385, "VAR1 Name"="Vd", "Decimal places in header"=i8 1, "VAR2 Name"="Vg") -> ("Header array"=w436:string[], "Data array"=w437:dbl[][])  [unwired: 14 in]
        n131 = call <userlib>:"4155C Write array to file.vi"("Byte Stream File Refnum"=w440, "Header"=w436, "Data Array"=w437, "error in (no error)"=w441) -> ("dup refnum"=w438:refnum<file>, "error out"=w439:errorcluster)  [unwired: 1 in]
        n132 = Close File(refnum=w438, error in=w439) -> (error out=w419:errorcluster)  [unwired: 1 out]
      }
      frame "output-fpp" {
        n133 = Number To Decimal String(number=w501) -> (decimal integer string=w502:string)  [unwired: 1 in]
        n134 = Bundle By Name(cluster=w477, "Emergency Stop"=w505) -> (w515:T6)
        n135 = Delete From Array(array=w492, index=0 ("Index")) -> (deleted portion=w490:string, array with subset deleted=w489:string[])  [unwired: 1 in]
        n136 = Concatenate Strings(w500, "-outputfpp-" ("Substring"), w502, ".txt" ("Substring")) -> (w504:string)
        n137 = VISA Write(VISA resource name=w468, write buffer=":PAGE:CHAN:MODE SWE;" ("write buffer (\"\")"), error in (no error)=w465) -> (VISA resource name out=w467:refnum<visa-resource-name>, error out=w466:errorcluster)  [unwired: 1 out]
        n138 = String To Path(string=w504) -> (path=w499:path)
        n139 = case shown="\"d\", Default" w490 {
          tunnel: [w516 w517] -> w488
          frame "s" {
            w516 = u16 0 items=["Single", "Double"] ("sweep mode")
          }
          frame "d", Default {
            w517 = u16 1 items=["Single", "Double"] ("sweep mode")
          }
        }
        n140 = Fract/Exp String To Number(string=w489) -> (number=w471:dbl[])  [unwired: 3 in, 1 out]
        n141 = Index Array(array=w471, index #1=0 ("Index")) -> (element #1=w487:dbl, element #2=w486:dbl, element #3=w485:dbl)  [unwired: 2 in]
        n142 = Delete From Array(array=w471, length=3 ("Length"), index=0 ("Index")) -> (array with subset deleted=w470:dbl[])  [unwired: 1 out]
        n143 = Bundle By Name(cluster=w479, "Gate Start"=w487, "Gate Stop"=w486, "Gate Step (linear only)"=w485, "Gate Compliance"=w497, "Range mode"=w463, "Range"=w462) -> (w514:T3)
        n144 = Index Array(array=w470, index #1=0 ("Index")) -> (element #1=w482:dbl, element #2=w481:dbl, element #3=w480:dbl)  [unwired: 2 in]
        n145 = call <vilib>:"compatOverwrite.vi"("overwrite (F)"=TRUE) -> ("overwrite?"=w450:T7)
        n146 = Bundle By Name(cluster=w478, "Drain Start"=w482, "Drain Stop"=w481, "Drain Step"=w480, "Drain Compliance"=w498, "Range mode"=w461, "Range"=w464) -> (w513:T4)
        n147 = call <userlib>:"4155C Output-FPP.vi"("VISA resource name in"=w467, "Gate"=w514, "Drain"=w513, "Timings"=w496, "error in (no error)"=w466, "sweep mode"=w488, "Panel controls"=w515) -> ("VD"=w455:dbl[], "Outparams"=w458:T8, "VISA Resource Name out"=w494:refnum<visa-resource-name>, "Vprobe2"=w454:dbl[], "ID"=w453:dbl[], "IG"=w452:dbl[], "Vprobe1"=w451:dbl[], "error out"=w495:errorcluster)  [unwired: 13 in]
        n148 = Unbundle By Name(w458) -> ("V2 Step"=w459:dbl, "V2 Start"=w457:dbl, "Number of points"=w456:i32)
        n149 = Open/Create/Replace File(file path (use dialog)=w499, error in=w495, operation (0:open)=w450) -> (refnum out=w510:refnum<file>, error out=w511:errorcluster)  [unwired: 3 in, 1 out]
        n150 = call <userlib>:"4155C Make Big 2d array FPP.vi"("1D Var1"=w455, "1d ID"=w453, "1d Vp2"=w454, "1d IG"=w452, "1d Vp1"=w451, "VAR2 START"=w457, "Number of VAR2 steps"=w456, "VAR2 STEP"=w459, "VAR1 Name"="Vd", "Decimal places in header"=i8 1, "VAR2 Name"="Vg") -> ("Header array"=w506:string[], "Data array"=w507:dbl[][])  [unwired: 15 in]
        n151 = call <userlib>:"4155C Write array to file.vi"("Byte Stream File Refnum"=w510, "Header"=w506, "Data Array"=w507, "error in (no error)"=w511) -> ("dup refnum"=w508:refnum<file>, "error out"=w509:errorcluster)  [unwired: 1 in]
        n152 = Close File(refnum=w508, error in=w509) -> (error out=w493:errorcluster)  [unwired: 1 out]
      }
      frame "itime" {
        n153 = Delete From Array(array=w531, index=0 ("Index")) -> (deleted portion=w532:string)  [unwired: 1 in, 1 out]
        n154 = case shown="\"l\"" w532 {
          tunnel: w530 -> [w536 w538 w541]
          tunnel: [w535 w537 w540] -> w523
          frame "s" {
            w534 = u32 0 items=["short  ", "medium  ", "long  "] ("integration time 2")
            n155 = Bundle By Name(cluster=w536, "integration time"=w534) -> (w535:T5)
          }
          frame "m", Default {
            w539 = u32 1 items=["short  ", "medium  ", "long  "] ("integration time 2")
            n156 = Bundle By Name(cluster=w538, "integration time"=w539) -> (w537:T5)
          }
          frame "l" {
            w542 = u32 2 items=["short  ", "medium  ", "long  "] ("integration time 2")
            n157 = Bundle By Name(cluster=w541, "integration time"=w542) -> (w540:T5)
          }
        }
      }
      frame "pulsed" {
        n158 = Delete From Array(array=w557, index=0 ("Index")) -> (deleted portion=w558:string, array with subset deleted=w545:string[])  [unwired: 1 in]
        n159 = case shown="\"on\", Default" w558 {
          tunnel: w556 -> [w568 w571]
          tunnel: [w567 w570] -> w549
          tunnel: w545 -> [w565 _]
          frame "on", Default {
            w566 = u16 1 items=["Continuous", "Pulsed"] ("sweep method")
            n160 = Fract/Exp String To Number(string=w565) -> (number=w563:dbl[])  [unwired: 3 in, 1 out]
            n161 = Index Array(array=w563, index #1=0 ("Index")) -> (element #1=w562:dbl, element #2=w561:dbl, element #3=w560:dbl)  [unwired: 2 in]
            n162 = Bundle By Name(cluster=w568, "sweep method"=w566, "Pulse period"=w562, "Base voltage"=w561, "Pulse width"=w560) -> (w567:T5)
          }
          frame "off" {
            w569 = u16 0 items=["Continuous", "Pulsed"] ("sweep method")
            n163 = Bundle By Name(cluster=w571, "sweep method"=w569) -> (w570:T5)
          }
        }
      }
      frame "gaterangemode" {
        n164 = Delete From Array(array=w584, index=0 ("Index")) -> (deleted portion=w585:string)  [unwired: 1 in, 1 out]
        n165 = case shown="\"f\"" w585 {
          tunnel: [w587 w588 w589] -> w574
          frame "a", Default {
            w587 = u16 0 items=["Auto", "Limited", "Fixed"] ("Gate Range\nmode 2")
          }
          frame "f" {
            w588 = u16 2 items=["Auto", "Limited", "Fixed"] ("Gate Range\nmode 2")
          }
          frame "l" {
            w589 = u16 1 items=["Auto", "Limited", "Fixed"] ("Gate Range\nmode 2")
          }
        }
      }
      frame "gaterange" {
        (unwired) u8 11 items=["10fA  ", "100fA  ", "1nA  ", "10nA", "100nA", "1uA", "10uA", "100uA", "1mA", "10mA", "100mA", "1A"] ("Gate Range 2")
        n166 = Delete From Array(array=w609, index=0 ("Index")) -> (deleted portion=w599:string)  [unwired: 1 in, 1 out]
        n167 = Scan Value(string=w599, format string="") -> (value=w597:dbl)  [unwired: 1 in, 1 out]
        n168 = Logarithm Base 10(1:w597) -> (0:w596:dbl)
        n169 = Round To Nearest(number=w596) -> (nearest integer value=w595:dbl)
        n170 = Add(x=w595, y=11.0) -> (x+y=w593:dbl)
        n171 = To Unsigned Byte Integer(number=w593) -> (unsigned 8bit integer=w592:u8)
      }
      frame "drainrange" {
        (unwired) u8 11 items=["10fA  ", "100fA  ", "1nA  ", "10nA", "100nA", "1uA", "10uA", "100uA", "1mA", "10mA", "100mA", "1A"] ("Gate Range 2")
        n172 = Delete From Array(array=w630, index=0 ("Index")) -> (deleted portion=w621:string)  [unwired: 1 in, 1 out]
        n173 = Scan Value(string=w621, format string="") -> (value=w619:dbl)  [unwired: 1 in, 1 out]
        n174 = Logarithm Base 10(1:w619) -> (0:w618:dbl)
        n175 = Round To Nearest(number=w618) -> (nearest integer value=w617:dbl)
        n176 = Add(x=w617, y=11.0) -> (x+y=w615:dbl)
        n177 = To Unsigned Byte Integer(number=w615) -> (unsigned 8bit integer=w614:u8)
      }
      frame "drainrangemode" {
        n178 = Delete From Array(array=w644, index=0 ("Index")) -> (deleted portion=w645:string)  [unwired: 1 in, 1 out]
        n179 = case shown="\"f\"" w645 {
          tunnel: [w647 w648 w649] -> w634
          frame "a", Default {
            w647 = u16 0 items=["Auto", "Limited", "Fixed"] ("Gate Range\nmode 2")
          }
          frame "f" {
            w648 = u16 2 items=["Auto", "Limited", "Fixed"] ("Gate Range\nmode 2")
          }
          frame "l" {
            w649 = u16 1 items=["Auto", "Limited", "Fixed"] ("Gate Range\nmode 2")
          }
        }
      }
      frame "Error", Default {
      }
      frame "logfile" {
        n180 = Number To Decimal String(number=w694) -> (decimal integer string=w698:string)  [unwired: 1 in]
        n181 = Concatenate Strings(w696, "logfile" ("Substring"), w698, ".txt" ("Substring")) -> (w693:string)
        n182 = String To Path(string=w693) -> (path=w666:path)
        n183 = Unbundle(w692) -> ("integration time"=w691:u32, "Short/Long integration time"=w690:dbl, "hold time (sec)"=w689:dbl, "delay time (sec)"=w688:dbl, "Step Time (0 disables)"=w687:dbl, "sweep method"=w686:u16, "Pulse period"=w685:dbl, "Base voltage"=w684:dbl, "Pulse width"=w683:dbl)
        n184 = Build Array(w691, w690, w689, w688, w687, w686, w685, w684, w683, w677, w678, w679, w680, w681, w682) -> (w670:dbl[])
        n185 = Insert Into Array(array=dbl[][] [] ("Input Array"), new element=w670) -> (w669:dbl[][])  [unwired: 2 in]
        n186 = call <vilib>:"compatOverwrite.vi"("overwrite (F)"=TRUE) -> ("overwrite?"=w664:T7)
        n187 = Open/Create/Replace File(file path (use dialog)=w666, error in=w668, operation (0:open)=w664) -> (refnum out=w674:refnum<file>, error out=w673:errorcluster)  [unwired: 3 in, 1 out]
        n188 = call <userlib>:"4155C Write array to file.vi"("Byte Stream File Refnum"=w674, "Header"=string[] ["Int Time", "Short/Long Itime", "Hold time", "Delay time", "Step time", "Sweep method", "Pulse period", "Base Voltage", "Pulse width", "Drain compliance", "Gate compliance", "Gate range mode", "Gate range", "S/D range mode", "S/D range"], "Data Array"=w669, "error in (no error)"=w673) -> ("dup refnum"=w676:refnum<file>, "error out"=w675:errorcluster)  [unwired: 1 in]
        n189 = Close File(refnum=w676, error in=w675) -> (error out=w667:errorcluster)  [unwired: 1 out]
      }
      frame "sample" {
        n190 = Number To Decimal String(number=w749) -> (decimal integer string=w748:string)  [unwired: 1 in]
        n191 = Fract/Exp String To Number(string=w745) -> (number=w705:dbl[])  [unwired: 3 in, 1 out]
        n192 = Concatenate Strings(w723, "-sample-" ("Substring"), w748, ".txt" ("Substring")) -> (w746:string)
        n193 = String To Path(string=w746) -> (path=w727:path)
        n194 = Index Array(array=w705, index=0 ("Index")) -> (element=w743:dbl)
        n195 = Index Array(array=w705, index=2 ("Index")) -> (element=w739:dbl)
        n196 = Index Array(array=w705, index=3 ("Index")) -> (element=w708:dbl)
        n197 = Index Array(array=w705, index=4 ("Index")) -> (element=w704:dbl)
        n198 = call <userlib>:"4155C Config Sampling Measurements.vi"("Sampling interval"=w704, "Sample time"=w708, "Display on/off"=TRUE, "Timings"=w714, "Num Points"=w739, "error in (no error)"=w751, "Drain Compliance"=w750, "Gate Compliance"=w724, "VISA session"=w752) -> ("error out"=w753:errorcluster, "dup VISA resource name"=w754:refnum<visa-resource-name>)  [unwired: 1 in]
        n199 = Index Array(array=w705, index=1 ("Index")) -> (element=w740:dbl)
        n200 = call <userlib>:"4155C Take Sample.vi"("Emergency Stop"=w720, "error in (no error)"=w753, "Vd"=w740, "Vg"=w743, "VISA resource name in"=w754) -> ("error out"=w718:errorcluster, "Id"=w756:dbl[], "Ig"=w729:dbl[], "VISA Resource Name out"=w716:refnum<visa-resource-name>, "Is"=w755:dbl[], "Time"=w733:dbl[])  [unwired: 1 in]
        n201 = Insert Into Array(array=dbl[][] [] ("Input Array"), new element=w733) -> (w732:dbl[][])  [unwired: 2 in]
        n202 = Insert Into Array(array=w732, new element=w729) -> (w731:dbl[][])  [unwired: 2 in]
        n203 = Insert Into Array(array=w731, new element=w756) -> (w730:dbl[][])  [unwired: 2 in]
        n204 = VISA Write(VISA resource name=w716, write buffer=":DISP ON" ("write buffer (\"\")"), error in (no error)=w718) -> (VISA resource name out=w715:refnum<visa-resource-name>, error out=w717:errorcluster)  [unwired: 1 out]
        n205 = Insert Into Array(array=w730, new element=w755) -> (w722:dbl[][])  [unwired: 2 in]
        n206 = Transpose 2D Array(2D array=w722) -> (transposed array=w721:dbl[][])
        n207 = call <vilib>:"compatOverwrite.vi"("overwrite (F)"=TRUE) -> ("overwrite?"=w702:T7)
        n208 = Open/Create/Replace File(file path (use dialog)=w727, error in=w717, operation (0:open)=w702) -> (refnum out=w736:refnum<file>, error out=w735:errorcluster)  [unwired: 3 in, 1 out]
        n209 = call <userlib>:"4155C Write array to file.vi"("Byte Stream File Refnum"=w736, "Header"=string[] ["Time /s", "Ig /A", "Id /A", "Is /A"], "Data Array"=w721, "error in (no error)"=w735) -> ("dup refnum"=w738:refnum<file>, "error out"=w737:errorcluster)  [unwired: 1 in]
        n210 = Close File(refnum=w738, error in=w737) -> (error out=w725:errorcluster)  [unwired: 1 out]
      }
      frame "samplei" {
        n211 = Number To Decimal String(number=w809) -> (decimal integer string=w808:string)  [unwired: 1 in]
        n212 = Fract/Exp String To Number(string=w805) -> (number=w771:dbl[])  [unwired: 3 in, 1 out]
        n213 = Concatenate Strings(w787, "-samplei-" ("Substring"), w808, ".txt" ("Substring")) -> (w806:string)
        n214 = String To Path(string=w806) -> (path=w790:path)
        n215 = Index Array(array=w771, index=4 ("Index")) -> (element=w765:dbl)
        n216 = Index Array(array=w771, index=3 ("Index")) -> (element=w766:dbl)
        n217 = Index Array(array=w771, index=1 ("Index")) -> (element=w768:dbl)
        n218 = Index Array(array=w771, index=0 ("Index")) -> (element=w769:dbl)
        n219 = Index Array(array=w771, index=2 ("Index")) -> (element=w767:dbl)
        n220 = call <userlib>:"4155C Config SamplingI Measurements.vi"("Sample time"=w767, "Display on/off"=TRUE, "Timings"=w779, "Num Points"=w768, "error in (no error)"=w811, "Sampling interval"=w766, "VISA session"=w812) -> ("error out"=w813:errorcluster, "dup VISA resource name"=w814:refnum<visa-resource-name>)  [unwired: 3 in]
        n221 = call <userlib>:"4155C Take SampleI.vi"("Emergency Stop"=w784, "error in (no error)"=w813, "Idg 2"=w769, "Vdg compliance 2"=w765, "VISA resource name in"=w814) -> ("error out"=w782:errorcluster, "Idg"=w816:dbl[], "Vdg"=w792:dbl[], "VISA Resource Name out"=w780:refnum<visa-resource-name>, "Is"=w815:dbl[], "Time"=w796:dbl[])  [unwired: 1 in]
        n222 = Insert Into Array(array=dbl[][] [] ("Input Array"), new element=w796) -> (w795:dbl[][])  [unwired: 2 in]
        n223 = Insert Into Array(array=w795, new element=w792) -> (w794:dbl[][])  [unwired: 2 in]
        n224 = Insert Into Array(array=w794, new element=w816) -> (w793:dbl[][])  [unwired: 2 in]
        n225 = VISA Write(VISA resource name=w780, write buffer=":DISP ON" ("write buffer (\"\")"), error in (no error)=w782) -> (VISA resource name out=w764:refnum<visa-resource-name>, error out=w781:errorcluster)  [unwired: 1 out]
        n226 = Insert Into Array(array=w793, new element=w815) -> (w786:dbl[][])  [unwired: 2 in]
        n227 = Transpose 2D Array(2D array=w786) -> (transposed array=w785:dbl[][])
        n228 = call <vilib>:"compatOverwrite.vi"("overwrite (F)"=TRUE) -> ("overwrite?"=w759:T7)
        n229 = Open/Create/Replace File(file path (use dialog)=w790, error in=w781, operation (0:open)=w759) -> (refnum out=w799:refnum<file>, error out=w798:errorcluster)  [unwired: 3 in, 1 out]
        n230 = call <userlib>:"4155C Write array to file.vi"("Byte Stream File Refnum"=w799, "Header"=string[] ["Time /s", "Vdg /V", "Idg /A", "Is /A"], "Data Array"=w785, "error in (no error)"=w798) -> ("dup refnum"=w801:refnum<file>, "error out"=w800:errorcluster)  [unwired: 1 in]
        n231 = Close File(refnum=w801, error in=w800) -> (error out=w762:errorcluster)  [unwired: 1 out]
        n232 = VISA Write(VISA resource name=w764, write buffer=";:PAGE:SCON:STAN OFF;:PAGE:CHAN:VSU2:DIS;" ("write buffer (\"\")"), error in (no error)=w762) -> (VISA resource name out=w760:refnum<visa-resource-name>, error out=w761:errorcluster)  [unwired: 1 out]
      }
      frame "#" {
        n233 = VISA Write(VISA resource name=w823, write buffer=":DISP ON" ("write buffer (\"\")"), error in (no error)=w822) -> (VISA resource name out=w821:refnum<visa-resource-name>, error out=w820:errorcluster)  [unwired: 1 out]
      }
      frame "stressV" {
        n234 = Number To Decimal String(number=w873) -> (decimal integer string=w872:string)  [unwired: 1 in]
        n235 = Fract/Exp String To Number(string=w869) -> (number=w841:dbl[])  [unwired: 3 in, 1 out]
        n236 = Concatenate Strings(w856, "-stressV-" ("Substring"), w872, ".txt" ("Substring")) -> (w870:string)
        n237 = String To Path(string=w870) -> (path=w860:path)
        n238 = Index Array(array=w841, index=3 ("Index")) -> (element=w838:dbl)
        n239 = Index Array(array=w841, index=1 ("Index")) -> (element=w836:dbl)
        n240 = Index Array(array=w841, index=0 ("Index")) -> (element=w835:dbl)
        n241 = Index Array(array=w841, index=4 ("Index")) -> (element=w840:dbl)
        n242 = Index Array(array=w841, index=2 ("Index")) -> (element=w837:dbl)
        n243 = call <userlib>:"4155C Config V Stress.vi"("VISA session"=w876, "ID compliance"=w838, "VD"=w836, "VG"=w835, "IG compliance"=w837, "error in (no error)"=w875, "Display on/off"=TRUE) -> ("dup VISA resource name"=w878:refnum<visa-resource-name>, "error out"=w877:errorcluster)
        n244 = call <userlib>:"4155C Apply Stress.vi"("error in (no error)"=w877, "Duration"=w840, "Emergency Stop"=w855, "VISA resource name in"=w878) -> ("error out"=w853:errorcluster, "VISA Resource Name out"=w851:refnum<visa-resource-name>)
        n245 = VISA Write(VISA resource name=w851, write buffer=":DISP ON" ("write buffer (\"\")"), error in (no error)=w853) -> (VISA resource name out=w850:refnum<visa-resource-name>, error out=w852:errorcluster)  [unwired: 1 out]
        n246 = call <vilib>:"compatOverwrite.vi"("overwrite (F)"=TRUE) -> ("overwrite?"=w834:T7)
        n247 = Open/Create/Replace File(file path (use dialog)=w860, error in=w852, operation (0:open)=w834) -> (refnum out=w863:refnum<file>, error out=w862:errorcluster)  [unwired: 3 in, 1 out]
        n248 = call <userlib>:"4155C Write array to file.vi"("Byte Stream File Refnum"=w863, "Header"=string[] ["V stress completed successfully", ""], "error in (no error)"=w862) -> ("dup refnum"=w865:refnum<file>, "error out"=w864:errorcluster)  [unwired: 2 in]
        n249 = Close File(refnum=w865, error in=w864) -> (error out=w858:errorcluster)  [unwired: 1 out]
      }
      frame "stressI" {
        n250 = Number To Decimal String(number=w916) -> (decimal integer string=w915:string)  [unwired: 1 in]
        n251 = Fract/Exp String To Number(string=w912) -> (number=w886:dbl[])  [unwired: 3 in, 1 out]
        n252 = Concatenate Strings(w899, "-stressI-" ("Substring"), w915, ".txt" ("Substring")) -> (w913:string)
        n253 = String To Path(string=w913) -> (path=w903:path)
        n254 = Index Array(array=w886, index=1 ("Index")) -> (element=w882:dbl)
        n255 = Index Array(array=w886, index=0 ("Index")) -> (element=w883:dbl)
        n256 = call <userlib>:"4155C Config I Stress.vi"("VISA session"=w919, "IDG"=w883, "VDG compliance"=w882, "error in (no error)"=w918, "Display on/off"=TRUE) -> ("dup VISA resource name"=w921:refnum<visa-resource-name>, "error out"=w920:errorcluster)
        n257 = Index Array(array=w886, index=2 ("Index")) -> (element=w884:dbl)
        n258 = call <userlib>:"4155C Apply Stress.vi"("error in (no error)"=w920, "Duration"=w884, "Emergency Stop"=w898, "VISA resource name in"=w921) -> ("error out"=w896:errorcluster, "VISA Resource Name out"=w894:refnum<visa-resource-name>)
        n259 = VISA Write(VISA resource name=w894, write buffer=":DISP ON" ("write buffer (\"\")"), error in (no error)=w896) -> (VISA resource name out=w893:refnum<visa-resource-name>, error out=w895:errorcluster)  [unwired: 1 out]
        n260 = call <vilib>:"compatOverwrite.vi"("overwrite (F)"=TRUE) -> ("overwrite?"=w881:T7)
        n261 = Open/Create/Replace File(file path (use dialog)=w903, error in=w895, operation (0:open)=w881) -> (refnum out=w906:refnum<file>, error out=w905:errorcluster)  [unwired: 3 in, 1 out]
        n262 = call <userlib>:"4155C Write array to file.vi"("Byte Stream File Refnum"=w906, "Header"=string[] ["I stress completed successfully", ""], "error in (no error)"=w905) -> ("dup refnum"=w908:refnum<file>, "error out"=w907:errorcluster)  [unwired: 2 in]
        n263 = Close File(refnum=w908, error in=w907) -> (error out=w901:errorcluster)  [unwired: 1 out]
      }
      frame "vsu2pulse" {
        n264 = Number To Decimal String(number=w957) -> (decimal integer string=w956:string)  [unwired: 1 in]
        n265 = Fract/Exp String To Number(string=w953) -> (number=w928:dbl[])  [unwired: 3 in, 1 out]
        n266 = Concatenate Strings(w941, "-vsu2-" ("Substring"), w956, ".txt" ("Substring")) -> (w954:string)
        n267 = String To Path(string=w954) -> (path=w945:path)
        n268 = Index Array(array=w928, index=1 ("Index")) -> (element=w927:dbl)
        n269 = Index Array(array=w928, index=0 ("Index")) -> (element=w925:dbl)
        n270 = call <userlib>:"4155C Config VSU2 Stress.vi"("error in (no error)"=w959, "VSU2"=w925, "Display on/off"=TRUE, "VISA session"=w960) -> ("error out"=w961:errorcluster, "dup VISA resource name"=w962:refnum<visa-resource-name>)
        n271 = call <userlib>:"4155C Apply Stress.vi"("error in (no error)"=w961, "Duration"=w927, "Emergency Stop"=w940, "VISA resource name in"=w962) -> ("error out"=w938:errorcluster, "VISA Resource Name out"=w936:refnum<visa-resource-name>)
        n272 = VISA Write(VISA resource name=w936, write buffer=":DISP ON" ("write buffer (\"\")"), error in (no error)=w938) -> (VISA resource name out=w935:refnum<visa-resource-name>, error out=w937:errorcluster)  [unwired: 1 out]
        n273 = call <vilib>:"compatOverwrite.vi"("overwrite (F)"=TRUE) -> ("overwrite?"=w924:T7)
        n274 = Open/Create/Replace File(file path (use dialog)=w945, error in=w937, operation (0:open)=w924) -> (refnum out=w948:refnum<file>, error out=w947:errorcluster)  [unwired: 3 in, 1 out]
        n275 = call <userlib>:"4155C Write array to file.vi"("Byte Stream File Refnum"=w948, "Header"=string[] ["VSU2 pulse completed successfully", ""], "error in (no error)"=w947) -> ("dup refnum"=w950:refnum<file>, "error out"=w949:errorcluster)  [unwired: 2 in]
        n276 = Close File(refnum=w950, error in=w949) -> (error out=w943:errorcluster)  [unwired: 1 out]
      }
      frame "sample-fpp" {
        w972 = string[] ["Time /s", "Id VgVd /A", "Ig VgVd /A", "Vp1 VgVd /V", "Vp2 VgVd /V"] ("Header")
        w976 = "%d" ("format string")
        n277 = Number To Decimal String(number=w1026) -> (decimal integer string=w1025:string)  [unwired: 1 in]
        n278 = Fract/Exp String To Number(string=w1022) -> (number=w1010:dbl[])  [unwired: 3 in, 1 out]
        n279 = Concatenate Strings(w1016, "-samplefpp-" ("Substring"), w1025, ".txt" ("Substring")) -> (w1023:string)
        n280 = String To Path(string=w1023) -> (path=w984:path)
        n281 = Index Array(array=w1010, index=0 ("Index")) -> (element=w970:dbl)
        n282 = Index Array(array=w1010, index=1 ("Index")) -> (element=w969:dbl)
        n283 = Index Array(array=w1010, index=2 ("Index")) -> (element=w1018:dbl)
        n284 = Index Array(array=w1010, index=3 ("Index")) -> (element=w1008:dbl)
        n285 = call <userlib>:"4155C Config Sampling Measurements FPP.vi"("VISA session"=w1029, "Num Points"=w1018, "Vg"=w970, "Display on/off"=TRUE, "Gate Compliance"=w1017, "Drain Compliance"=w1027, "Standby"="Standby", "error in (no error)"=w1028, "Timings"=w1015, "Vd"=w969, "Sample time"=w1008) -> ("dup VISA resource name"=w986:refnum<visa-resource-name>, "error out"=w985:errorcluster)  [unwired: 3 in]
        n286 = Number To Decimal String(number=w970) -> (decimal integer string=w996:string)  [unwired: 1 in]
        n287 = call <userlib>:"4155C Take Sample FPP.vi"("VISA resource name in"=w986, "error in (no error)"=w985, "Emergency Stop"=w987) -> ("Time"=w991:dbl[], "Vp1"=w1001:dbl[], "VISA Resource Name out"=w967:refnum<visa-resource-name>, "Ig"=w989:dbl[], "Id"=w990:dbl[], "Vp2"=w999:dbl[], "error out"=w988:errorcluster)  [unwired: 10 in]
        n288 = Insert Into Array(array=dbl[][] [] ("Input Array"), new element=w991) -> (w1005:dbl[][])  [unwired: 2 in]
        n289 = Number To Decimal String(number=w969) -> (decimal integer string=w994:string)  [unwired: 1 in]
        n290 = Insert Into Array(array=w1005, new element=w990) -> (w1004:dbl[][])  [unwired: 2 in]
        n291 = Concatenate Strings("(Vg = " ("Substring"), w996, "V, Vd = " ("Substring"), w994, "V)" ("Substring")) -> (w992:string)
        n292 = Insert Into Array(array=w1004, new element=w989) -> (w1003:dbl[][])  [unwired: 2 in]
        n293 = Insert Into Array(array=w1003, new element=w1001) -> (w1000:dbl[][])  [unwired: 2 in]
        n294 = Insert Into Array(array=w1000, new element=w999) -> (w968:dbl[][])  [unwired: 2 in]
        n295 = call <vilib>:"compatOverwrite.vi"("overwrite (F)"=TRUE) -> ("overwrite?"=w965:T7)
        n296 = Open/Create/Replace File(file path (use dialog)=w984, error in=w988, operation (0:open)=w965) -> (refnum out=w981:refnum<file>, error out=w982:errorcluster)  [unwired: 3 in, 1 out]
        n297 = Array To Spreadsheet String(array=w972, 3:w976) -> (spreadsheet string=w978:string)  [unwired: 1 in]
        n298 = Transpose 2D Array(2D array=w968) -> (transposed array=w998:dbl[][])
        n299 = Search and Replace String(replace all?=TRUE ("replace all? (F)"), input string=w978, search string="VgVd", replace string=w992) -> (result string=w974:string)  [unwired: 4 in, 3 out]
        n300 = Spreadsheet String To Array(format string=w976, spreadsheet string=w974, array type (2D Dbl)=w972) -> (array=w973:string[])  [unwired: 1 in]
        n301 = call <userlib>:"4155C Write array to file.vi"("Byte Stream File Refnum"=w981, "Header"=w973, "Data Array"=w998, "error in (no error)"=w982) -> ("dup refnum"=w979:refnum<file>, "error out"=w980:errorcluster)  [unwired: 1 in]
        n302 = Close File(refnum=w979, error in=w980) -> (error out=w966:errorcluster)  [unwired: 1 out]
      }
      frame "resample-fpp" {
        w1041 = string[] ["Time /s", "Id VgVd /A", "Ig VgVd /A", "Vp1 VgVd /V", "Vp2 VgVd /V"] ("Header")
        w1045 = "%d" ("format string")
        n303 = Number To Decimal String(number=w1087) -> (decimal integer string=w1086:string)  [unwired: 1 in]
        n304 = Fract/Exp String To Number(string=w1083) -> (number=w1034:dbl[])  [unwired: 3 in, 1 out]
        n305 = Concatenate Strings(w1079, "-resamplefpp-" ("Substring"), w1086, ".txt" ("Substring")) -> (w1084:string)
        n306 = String To Path(string=w1084) -> (path=w1053:path)
        n307 = Index Array(array=w1034, index=0 ("Index")) -> (element=w1040:dbl)
        n308 = Index Array(array=w1034, index=1 ("Index")) -> (element=w1039:dbl)
        n309 = Number To Decimal String(number=w1040) -> (decimal integer string=w1063:string)  [unwired: 1 in]
        n310 = call <userlib>:"4155C Take Sample FPP.vi"("VISA resource name in"=w1036, "error in (no error)"=w1035, "Emergency Stop"=w1054) -> ("Time"=w1058:dbl[], "Vp1"=w1068:dbl[], "VISA Resource Name out"=w1038:refnum<visa-resource-name>, "Ig"=w1056:dbl[], "Id"=w1057:dbl[], "Vp2"=w1066:dbl[], "error out"=w1055:errorcluster)  [unwired: 10 in]
        n311 = Insert Into Array(array=dbl[][] [] ("Input Array"), new element=w1058) -> (w1072:dbl[][])  [unwired: 2 in]
        n312 = Number To Decimal String(number=w1039) -> (decimal integer string=w1061:string)  [unwired: 1 in]
        n313 = Insert Into Array(array=w1072, new element=w1057) -> (w1071:dbl[][])  [unwired: 2 in]
        n314 = Concatenate Strings("(Vg = " ("Substring"), w1063, "V, Vd = " ("Substring"), w1061, "V)" ("Substring")) -> (w1059:string)
        n315 = Insert Into Array(array=w1071, new element=w1056) -> (w1070:dbl[][])  [unwired: 2 in]
        n316 = Insert Into Array(array=w1070, new element=w1068) -> (w1067:dbl[][])  [unwired: 2 in]
        n317 = Insert Into Array(array=w1067, new element=w1066) -> (w1033:dbl[][])  [unwired: 2 in]
        n318 = call <vilib>:"compatOverwrite.vi"("overwrite (F)"=TRUE) -> ("overwrite?"=w1032:T7)
        n319 = Open/Create/Replace File(file path (use dialog)=w1053, error in=w1055, operation (0:open)=w1032) -> (refnum out=w1050:refnum<file>, error out=w1051:errorcluster)  [unwired: 3 in, 1 out]
        n320 = Array To Spreadsheet String(array=w1041, 3:w1045) -> (spreadsheet string=w1047:string)  [unwired: 1 in]
        n321 = Transpose 2D Array(2D array=w1033) -> (transposed array=w1065:dbl[][])
        n322 = Search and Replace String(replace all?=TRUE ("replace all? (F)"), input string=w1047, search string="VgVd", replace string=w1059) -> (result string=w1043:string)  [unwired: 4 in, 3 out]
        n323 = Spreadsheet String To Array(format string=w1045, spreadsheet string=w1043, array type (2D Dbl)=w1041) -> (array=w1042:string[])  [unwired: 1 in]
        n324 = call <userlib>:"4155C Write array to file.vi"("Byte Stream File Refnum"=w1050, "Header"=w1042, "Data Array"=w1065, "error in (no error)"=w1051) -> ("dup refnum"=w1048:refnum<file>, "error out"=w1049:errorcluster)  [unwired: 1 in]
        n325 = Close File(refnum=w1048, error in=w1049) -> (error out=w1037:errorcluster)  [unwired: 1 out]
      }
    }
    n326 = local write "Lines left to run:"(w49) -> ()
    n327 = Empty String/Path?(string/path=w49) -> (empty?=w85:bool)
    n328 = Not(x=w85) -> (.not. x?=w84:bool)
  }
  "error out" <- w1
